vi "Send BackupDB - Timed.vi"(5 "# Copies (0 = infinite repeat)":u32=1, 6 "Milliseconds To Wait":i32=1000, 7 "Message Priority (Normal)":T1=enum."Normal", 8 "error in (no error)":errorcluster, 11 "Message Enqueuer":refnum<class "Message Enqueuer.lvclass">) -> (0 "error out":errorcluster, 2 "Delivery Notifier":refnum<notifier>, 3 "Message Enqueuer out":refnum<class "Message Enqueuer.lvclass">)   [LabVIEW 2014, in "TableLogger_Actor.lvlib" / "BackupDB Msg.lvclass"]
doc: "This VI sends the message to an actor."
uses:
  BackupDB Msg.lvclass
  <vilib>/ActorFramework/Message Enqueuer/Message Enqueuer.lvclass
  <vilib>/ActorFramework/Message Enqueuer/Message Priority.ctl
  <vilib>/ActorFramework/Time-Delayed Send Message/Time-Delay Override Options.ctl
panel:
  # "Connector Pane"
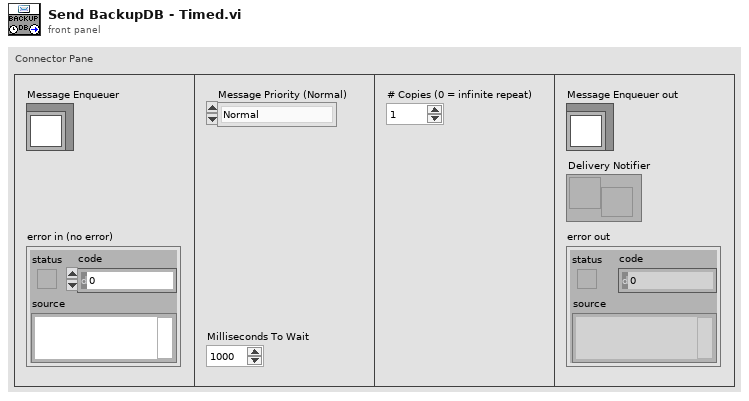
[diagram p1: front panel]
types:
  T1 = typedef "Actor Framework.lvlib/Message Enqueuer.lvclass/Message Priority.ctl" = enum16{"Low", "Normal", "High"}
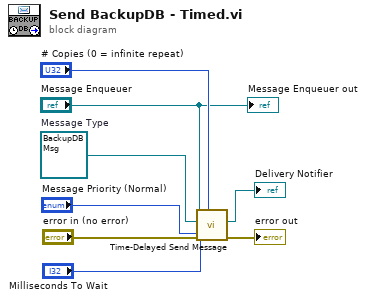
[diagram p0: block diagram]
diagram:
  w6 = refnum<class "BackupDB Msg.lvclass"> refnum  # Message Type
  n1 = call <vilib>:"Time-Delayed Send Message.vi"("Message Priority (Normal)"="Message Priority (Normal)", "# Copies (0 = infinite repeat)"="# Copies (0 = infinite repeat)", "error in (no error)"="error in (no error)", "Milliseconds To Wait"="Milliseconds To Wait", "Message"=w6, "Message Enqueuer"="Message Enqueuer") -> ("error out"=→"error out":errorcluster, "Delivery Notifier"=→"Delivery Notifier":refnum<notifier>)  [unwired: 4 in]
  "Message Enqueuer out" <- "Message Enqueuer"
